vi "OnceOnPress.vi"(1 "Button In":bool) -> (0 "Value Out":bool)   [LabVIEW 2018]
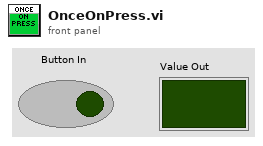
[diagram p1: front panel]
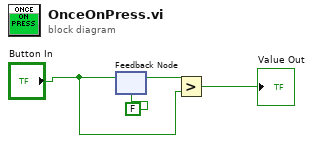
[diagram p0: block diagram]
diagram:
  n1 = feedback #1(FALSE) -> (w4:bool)
  n2 = feedback-in #1("Button In") -> ()
  n3 = Greater?(x=w4, y="Button In") -> (0:→"Value Out":bool)
